vi "Suma.vi"(2 "PORT":refnum<visa-resource-name>, 3 "Y":dbl, 4 "X":dbl) -> (1 "SUMA":dbl)   [LabVIEW 2019]
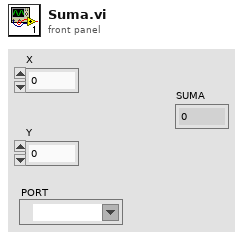
[diagram p1: front panel]
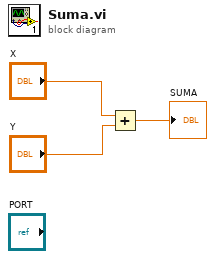
[diagram p0: block diagram]
diagram:
  n1 = Add(x="X", y="Y") -> (x+y=→"SUMA":dbl)
